vi "ReceiveMessages.vi"(6 "timeout(100)":i32=100, 8 "error in (no error)":errorcluster, 9 "priority action":string, 10 "default action":string, 11 "qbus in":refnum<class "Qbus.lvclass">) -> (0 "error out":errorcluster, 1 "message value":variant, 2 "action":string, 3 "qbus out":refnum<class "Qbus.lvclass">, 4 "exit":bool)   [LabVIEW 2017, in "TraceLogger.lvlib"]
uses:
  <vilib>/addons/TraceLogger/TraceLogger.lvlib
  <vilib>/addons/Qbus/Qbus.lvclass
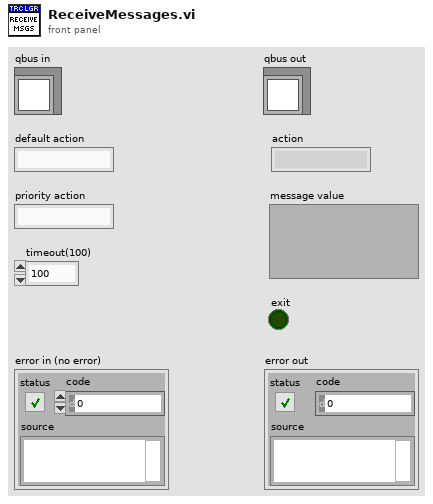
[diagram p1: front panel]
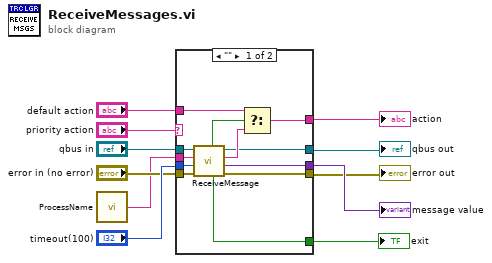
[diagram p0: block diagram]
diagram:
  n1 = call <vilib>:"ProcessName.vi"() -> ("process name"=w2:string)  [unwired: 5 in]
  n2 = case shown="\"\"" "priority action" {
    selector: "priority action" -> [_ w24]
    tunnel: "error in (no error)" -> [w14 w26]
    tunnel: [w20 w26] -> w7
    tunnel: [w19 _] -> w9
    tunnel: [w15 _] -> w4
    tunnel: "default action" -> [w23 _]
    tunnel: [w22 w24] -> w1
    tunnel: [w17 w25] -> w8
    tunnel: "timeout(100)" -> [w13 _]
    tunnel: "qbus in" -> [w16 w25]
    tunnel: w2 -> [w12 _]
    frame "" {
      n3 = call <vilib>:"ReceiveMessage.vi"("error in (no error)"=w14, "timeout (0)"=w13, "process name"=w12, "Qbus in"=w16) -> ("error in (no error)"=w20:errorcluster, "message value"=w19:variant, "message name"=w18:string, "Qbus out"=w17:refnum<class "Qbus.lvclass">, "exit"=w15:bool, "timed out"=w21:bool)  [unwired: 2 in]
      n4 = Select(t=w23, s=w21, f=w18) -> (s? t:f=w22:string)
    }
    frame Default {
    }
  }
  "message value" <- w9
  "action" <- w1
  "qbus out" <- w8
  "error out" <- w7
  "exit" <- w4
